vi "Write p2.vi"(8 "error in (no error)":errorcluster, 10 "p2":u16, 11 "CameraSession in":refnum<class "CameraSession.lvclass">) -> (0 "error out":errorcluster, 3 "CameraSession out":refnum<class "CameraSession.lvclass">)   [LabVIEW 2013, in "CameraSession.lvclass"]
uses:
  CameraSession.lvclass
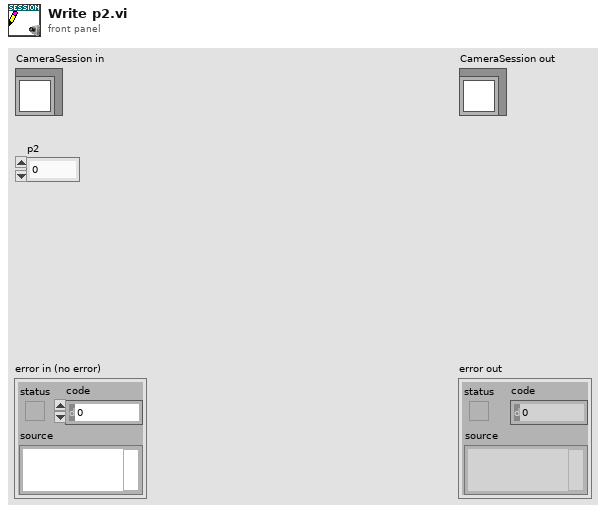
[diagram p1: front panel]
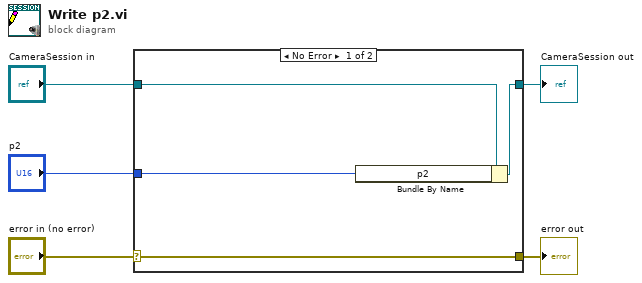
[diagram p0: block diagram]
diagram:
  n1 = case shown="No Error" "error in (no error)" {
    selector: "error in (no error)" -> [w9 w10]
    tunnel: [w9 w10] -> w4
    tunnel: [w7 w11] -> w2
    tunnel: "CameraSession in" -> [w8 w11]
    tunnel: "p2" -> [w6 _]
    frame No Error {
      n2 = Bundle By Name(cluster=w8, "p2"=w6) -> (w7:refnum<class "CameraSession.lvclass">)
    }
    frame Error {
    }
  }
  "error out" <- w4
  "CameraSession out" <- w2
